vi "Submit.vi"(0 "CommitNIPKG_LV in":refnum<class "CommitNIPKG_LV.lvclass">, 5 "Export":refnum<class "Export.lvclass">, 11 "error in (no error)":errorcluster) -> (4 "CommitNIPKG_LV out":refnum<class "CommitNIPKG_LV.lvclass">, 15 "error out":errorcluster)   [LabVIEW 2017, in "CL_G3_VIComponentBuilder.lvlib" / "CommitNIPKG_LV.lvclass"]
doc: "Performs the submit operations for this export."
uses:
  CommitNIPKG_LV.lvclass
  C:/Tool Chain Support/Software Module Builder/Source/Commit Behavior/Commit/Commit.lvclass
  Exports/Exports/Export.lvclass
  Exports/NIPKG_LV/NIPKG_LV.lvclass
  C:/Tool Chain Support/Software Module Builder/Source/Exports/Exports/Export.lvclass
  Exports/Exports/Export.lvclass/Export.ctl
  CommitNIPKG_LV.lvclass/CommitNIPKG_LV.ctl
  Commit/Commit.lvclass/Commit.ctl
  Exports/Exports/Accessors/Read Built Export's Full Path.vi
  Accessors/Read Commit Feed Folderpaths.vi
  Commit/Accessors/Read Exports Commit Destination Folder.vi
  <userlib>/_Cirrus Logic/NI Package Manager API/Source/TCS_NIPKG_API.lvlib
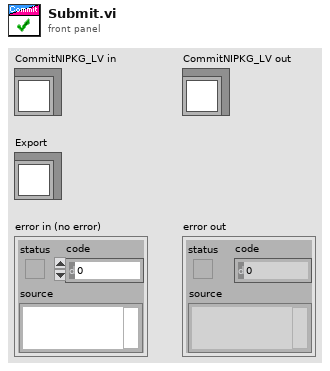
[diagram p1: front panel]
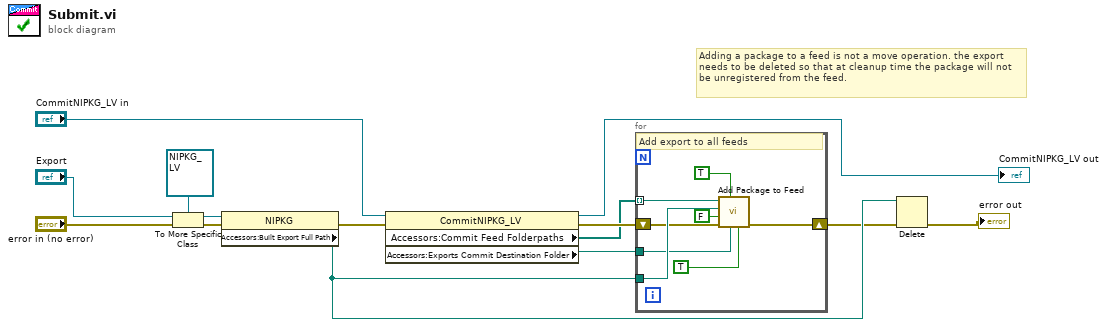
[diagram p0: block diagram]
diagram:
  # "Adding a package to a feed is not a move operation. the export needs to be deleted so that at cleanup time the package will not be unregistered from the feed."
  n1 = To More Specific Class(target class=refnum<class "NIPKG_LV.lvclass"> refnum ("CL_G3_VIComponentBuilder.lvlib:NIPKG"), reference="Export", error in="error in (no error)") -> (specific class reference=w9:refnum<class "NIPKG_LV.lvclass">, error out=w11:errorcluster)
  n2 = property class="NIPKG"(reference=w9, error in=w11) -> (error out=w10:errorcluster, "Accessors:Built Export Full Path"=w3:path)  [unwired: 1 out]
  n3 = property class="CommitNIPKG_LV"(reference="CommitNIPKG_LV in", error in=w10) -> (reference out=→"CommitNIPKG_LV out":refnum<class "CommitNIPKG_LV.lvclass">, error out=w7:errorcluster, "Accessors:Commit Feed Folderpaths"=w6:path[], "Accessors:Exports Commit Destination Folder"=w5:path)
  n4 = for {
    tunnel: w3 -> [w22]
    shift-right: [w20] -> w2
    shift-left: w7 -> [w21]
    tunnel: w6 -> [w19] mode=indexing
    tunnel: w5 -> [w18]
    # "Add export to all feeds"
    n5 = call <userlib>:"Add Package to Feed.vi"("create new package destination folderpath if none exists (F)"=TRUE, "package destination folderpath"=w18, "create new feed if none exists (F)"=TRUE, "error in"=w21, "overwrite existing package (T)"=FALSE, "package source filepath"=w22, "feed folderpath"=w19) -> ("error out"=w20:errorcluster)  [unwired: 4 in]
  }
  n6 = Delete(path (use dialog)=w3, error in=w2) -> (error out=→"error out":errorcluster)  [unwired: 3 in, 2 out]
